vi "Send Query Instruments.vi"(7 "Message Priority (Normal)":T1=enum."Normal", 8 "error in (no error)":errorcluster, 10 "Instrument Notifier":refnum<notifier>, 11 "Message Enqueuer":refnum<class "Message Enqueuer.lvclass">) -> (0 "error out":errorcluster, 3 "Message Enqueuer out":refnum<class "Message Enqueuer.lvclass">)   [LabVIEW 2019, in "Base Software.lvlib" / "Main.lvlib" / "Query Instruments Msg.lvclass"]
doc: "This VI sends the message to an actor."
uses:
  Query Instruments Msg.lvclass
  builds/Engine/Actor Framework.lvlibp/1abvi3w/vi.lib/ActorFramework/Message Enqueuer/Message Enqueuer.lvclass
  builds/Engine/Actor Framework.lvlibp/1abvi3w/vi.lib/ActorFramework/Message Enqueuer/Message Priority.ctl
  Query Instruments Msg.lvclass/Query Instruments Msg.ctl
  C:/Users/Public/Documents/Development/builds/Engine/Actor Framework.lvlibp/1abvi3w/vi.lib/ActorFramework/Message/Message.lvclass
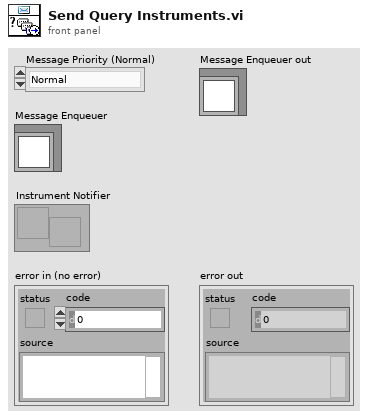
[diagram p1: front panel]
types:
  T1 = typedef "Actor Framework.lvlibp/Message Enqueuer.lvclass/Message Priority.ctl" = enum16{"Low", "Normal", "High"}
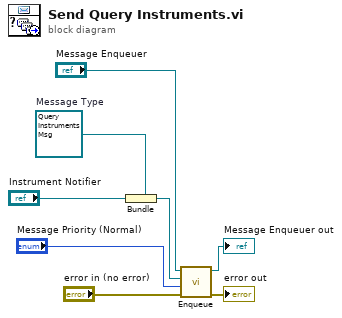
[diagram p0: block diagram]
diagram:
  w5 = refnum<class "Query Instruments Msg.lvclass"> refnum  # Message Type
  n1 = Bundle(cluster=w5, "Instrument Notifier") -> (w4:refnum<class "Query Instruments Msg.lvclass">)
  n2 = call "Enqueue.vi"("error in (no error)"="error in (no error)", "Message Priority (Normal)"="Message Priority (Normal)", "Message"=w4, "Message Enqueuer in"="Message Enqueuer") -> ("error out"=→"error out":errorcluster, "Message Enqueuer out"=→"Message Enqueuer out":refnum<class "Message Enqueuer.lvclass">)  [unwired: 6 in]
